vi "ziModGetHeader.vi"   [LabVIEW 2009, in "Zurich Instruments LabOne.lvlib"]
uses:
  <instrlib>/Zurich Instruments LabOne/Zurich Instruments LabOne.lvlib
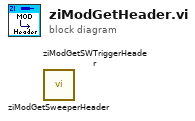
[diagram p0: block diagram]
diagram:
  n1 = call <instrlib>:"ziModGetSweeperHeader.vi"() -> ()  [unwired: 9 in, 3 out]
  n2 = call <instrlib>:"ziModGetSWTriggerHeader.vi"() -> ()  [unwired: 9 in, 3 out]
